vi "BoltekOutStr.vi"(0 "noise?":bool, 2 "+ or -":bool=TRUE, 3 "badFormat?":bool, 4 "inputs_constant?":bool, 5 "Kv/m Amplitude":dbl format="%.2f", 6 "constant":dbl, 7 "seconds since 1Jan1904":dbl format="%.2f") -> (1 "String Boltek":string)   [LabVIEW 2010]
panel:
  out "data string":string
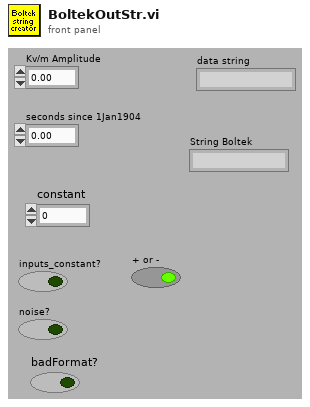
[diagram p1: front panel]
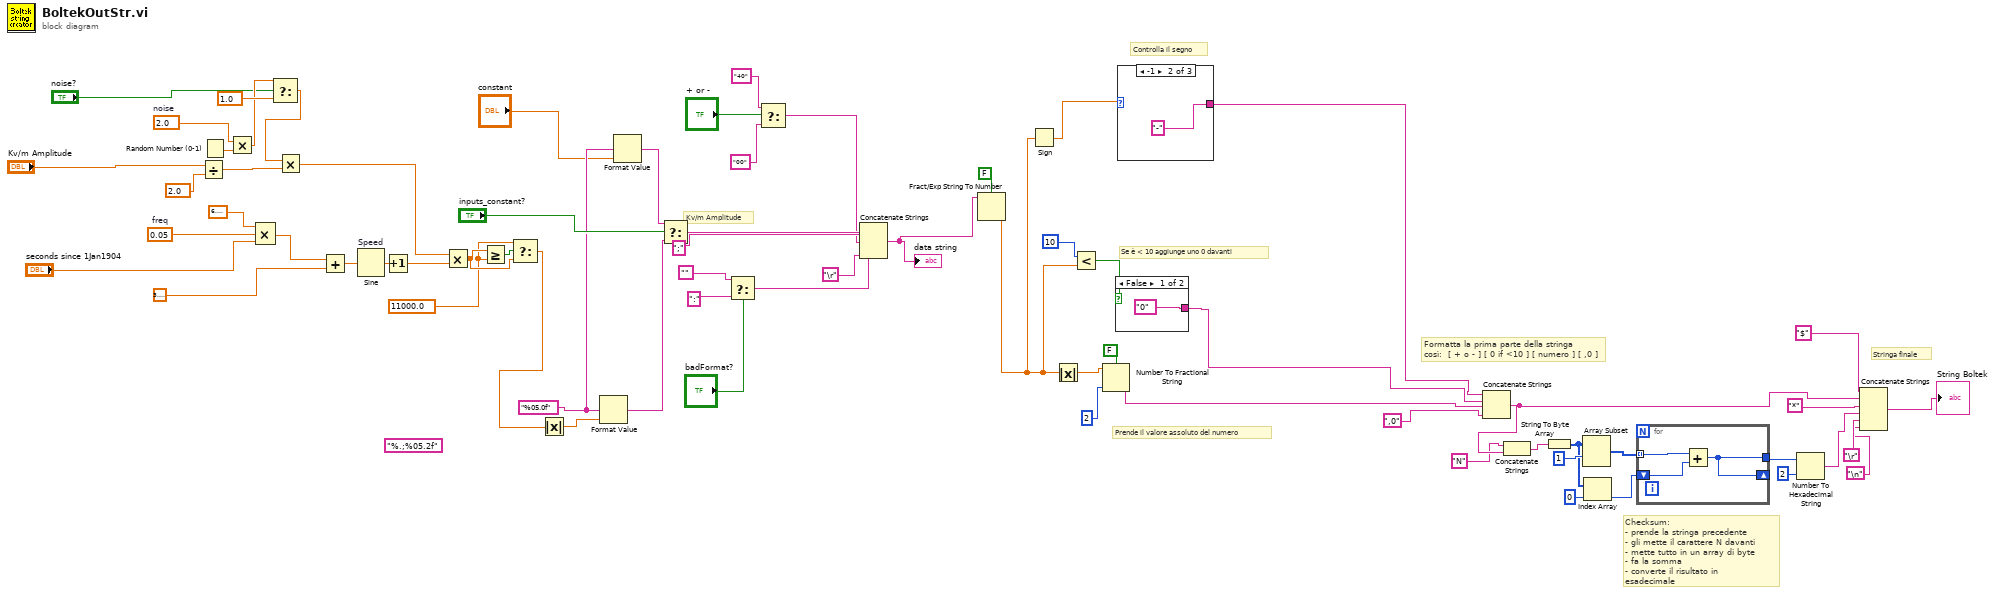
[diagram p0: block diagram]
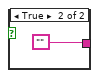
[diagram p2: hidden frame]
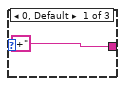
[diagram p3: hidden frame]
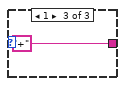
[diagram p4: hidden frame]
diagram:
  (unwired) "%.;%05.2f" ("format string")
  w13 = "%05.0f" ("format string")
  w30 = 2.0  # noise
  w31 = 0.05  # freq
  w39 = 11000.0 ("y")
  # "Kv/m Amplitude"
  # "Stringa finale"
  # "Checksum:\n- prende la stringa precedente\n- gli mette il carattere N davanti\n- mette tutto in un array di byte\n- fa la somma\n- converte il risultato in esadecimale"
  # "Formatta la prima parte della stringa\ncosì:  [ + o - ] [ 0 if <10 ] [ numero ] [ ,0 ]"
  # "Prende il valore assoluto del numero"
  # "Se è < 10 aggiunge uno 0 davanti"
  # "Controlla il segno"
  n1 = Divide(x="Kv/m Amplitude", y=2.0) -> (x/y=w35:dbl)
  n2 = Random Number (0-1)() -> (number: 0 to 1=w29:dbl)
  n3 = Multiply(x=w30, y=w29) -> (x*y=w20:dbl)
  n4 = Compound Arithmetic op=MULTIPLY(6.283185307179586, w31, "seconds since 1Jan1904") -> (w27:dbl)
  n5 = Select(t=w20, s="noise?", f=1.0) -> (s? t:f=w21:dbl)
  n6 = Multiply(x=w21, y=w35) -> (x*y=w37:dbl)
  n7 = Add(x=w27, y=3.141592653589793) -> (x+y=w26:dbl)
  n8 = Sine "Speed"(x=w26) -> (sin(x)=w25:dbl)
  n9 = Increment(x=w25) -> (x+1=w34:dbl)
  n10 = Multiply(x=w37, y=w34) -> (x*y=w40:dbl)
  n11 = Greater Or Equal?(x=w40, y=w39) -> (x >= y?=w38:bool)
  n12 = Select(t=w39, s=w38, f=w40) -> (s? t:f=w16:dbl)
  n13 = Absolute Value(x=w16) -> (abs(x)=w15:dbl)
  n14 = Format Value(format string=w13, value (0)=w15) -> (output string=w17:string)  [unwired: 1 in]
  n15 = Format Value(format string=w13, value (0)="constant") -> (output string=w11:string)  [unwired: 1 in]
  n16 = Select(t=w11, s="inputs_constant?", f=w17) -> (s? t:f=w18:string)
  n17 = Select(t="", s="badFormat?", f=":" ("string")) -> (s? t:f=w7:string)
  n18 = Select(t="40" ("string"), s="+ or -", f="00" ("string")) -> (s? t:f=w2:string)
  n19 = Concatenate Strings(w18, ";" ("string"), w2, w7, "\r") -> (w1:string)
  "data string" <- w1
  n20 = Fract/Exp String To Number(use system decimal point (T)=FALSE, string=w1) -> (number=w59:dbl)  [unwired: 2 in, 1 out]
  n21 = Sign(1:w59) -> (0:w68:dbl)
  n22 = Absolute Value(x=w59) -> (abs(x)=w58:dbl)
  n23 = Less?(x=10, y=w59) -> (x < y?=w61:bool)
  n24 = Number To Fractional String(use system decimal point (T)=FALSE, number=w58, precision (6)=2) -> (F-format string=w64:string)  [unwired: 1 in]
  n25 = case shown="False" w61 {
    tunnel: ["0" ""] -> w60
    frame False {
    }
    frame True {
    }
  }
  n26 = case shown="-1" w68 {
    tunnel: ["+" "-" "+"] -> w44
    frame 0, Default {
    }
    frame -1 {
    }
    frame 1 {
    }
  }
  n27 = Concatenate Strings(w44, w60, w64, ",0") -> (w43:string)
  n28 = Concatenate Strings("N", w43) -> (w41:string)
  n29 = String To Byte Array(string=w41) -> (unsigned byte array=w55:u8[])
  n30 = Array Subset(array=w55, index=1) -> (w57:u8[])  [unwired: 1 in]
  n31 = Index Array(array=w55, index=0) -> (element=w53:u8)
  n32 = for {
    tunnel: w57 -> [w76] mode=indexing
    shift-right: [w74] -> _
    shift-left: w53 -> [w75]
    tunnel: [w74] -> w52
    n33 = Add(x=w76, y=w75) -> (x+y=w74:u8)
  }
  n34 = Number To Hexadecimal String(1:i16 2 ("width (-)"), 2:w52) -> (0:w50:string)
  n35 = Concatenate Strings("$", w43, "*", w50, "\r", "\n") -> (→"String Boltek":string)
